vi "NXT_HINDBRAIN Move Motors.vi"(0 "NXT":T3, 1 "Motor Disable":bool, 2 "Tugboat Properties":T1={"_name"="Enterprise", "_pitch"=440, "_rudderCenter"=1450, "_propCenter"=1000, "_irServoCenter"=1000, "_rudderMin"=1450, "_rudderMax"=1450, "_propMin"=1000, "_propMax"=1000, "_irServoMin"=1000, "_irServoMax"=1000}, 3 "_motorData":T2) -> ()   [LabVIEW 2012, in "Tugboat.lvrbt"]
uses:
  Tugboat.lvrbt
  <vilib>/NXT/Subs/LVHSConnector.ctl
  motorData_t.ctl
  tugProperties_t.ctl
  <vilib>/NXT/Block Support/NXT_InputPort.ctl
  <vilib>/NXT/Dual Mode Library/prims/inRangeAndCoerce/inRangeAndCoerce_int.vi
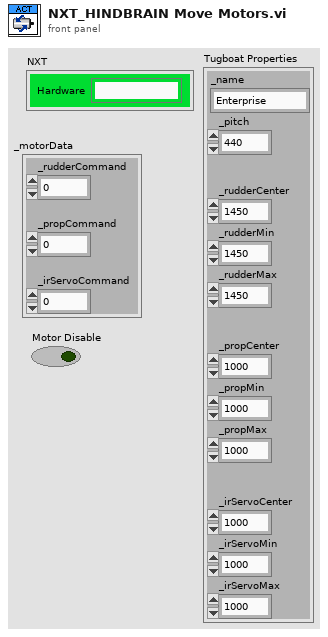
[diagram p1: front panel]
types:
  T1 = typedef "tugProperties_t.ctl" = cluster{"_name":string, "_pitch":i32, "_rudderCenter":u16, "_propCenter":u16, "_irServoCenter":u16, "_rudderMin":u16, "_rudderMax":u16, "_propMin":u16, "_propMax":u16, "_irServoMin":u16, "_irServoMax":u16}
  T2 = typedef "motorData_t.ctl" = cluster{"_rudderCommand":u16, "_propCommand":u16, "_irServoCommand":u16}
  T3 = typedef "LVHSConnector.ctl" = cluster{"Hardware":string, "Flattened String":string}
  T4 = cluster{"Servo Number":u8, "Position":u16, "Speed":u8}
  T5 = typedef "NXT_InputPort.ctl" = u8
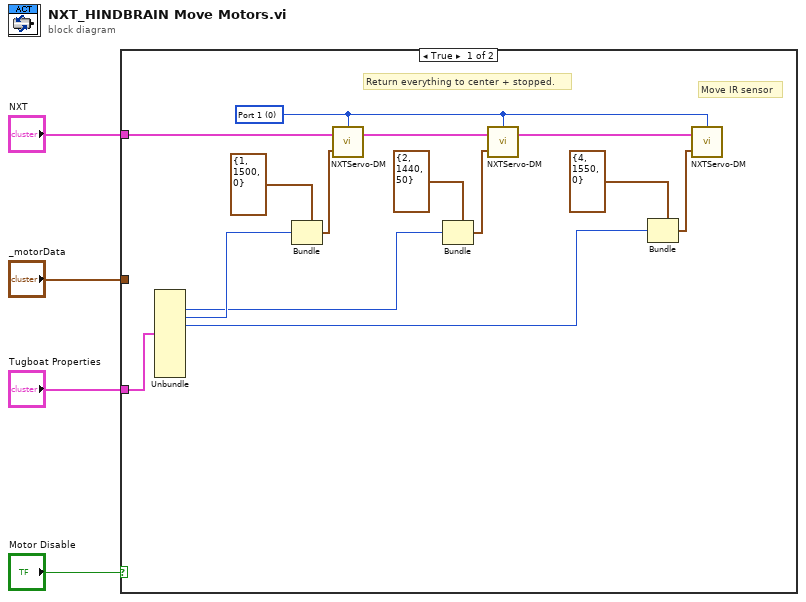
[diagram p0: block diagram]
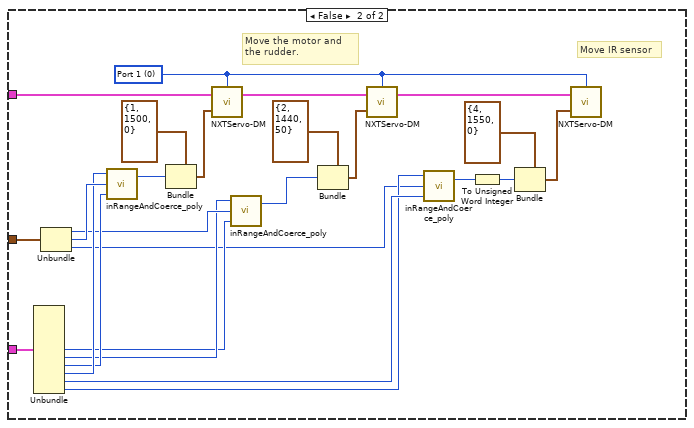
[diagram p2: hidden frame]
diagram:
  n1 = case shown="True" "Motor Disable" {
    tunnel: "NXT" -> [w15 w36]
    tunnel: "_motorData" -> [_ w35]
    tunnel: "Tugboat Properties" -> [w13 w31]
    frame True {
      w16 = T5 0 items=["Port 1", "Port 2", "Port 3", "Port 4"] ("Input Port")
      # "Move IR sensor"
      # "Return everything to center + stopped."
      n2 = Unbundle(w13) -> ("_rudderCenter"=w8:u16, "_propCenter"=w12:u16, "_irServoCenter"=w5:u16)  [unwired: 8 out]
      n3 = Bundle(cluster=T4 {"Servo Number"=1, "Position"=1500, "Speed"=0} ("Input of NXTServo"), "Position"=w12) -> (w11:T4)  [unwired: 2 in]
      n4 = call "NXTServo-DM.vi"("Input of NXTServo"=w11, "NXT"=w15, "Input Port"=w16) -> ("NXT dup"=w18:T3)  [unwired: 1 out]
      n5 = Bundle(cluster=T4 {"Servo Number"=2, "Position"=1440, "Speed"=50} ("Input of NXTServo"), "Position"=w8) -> (w9:T4)  [unwired: 2 in]
      n6 = call "NXTServo-DM.vi"("Input of NXTServo"=w9, "NXT"=w18, "Input Port"=w16) -> ("NXT dup"=w17:T3)  [unwired: 1 out]
      n7 = Bundle(cluster=T4 {"Servo Number"=4, "Position"=1550, "Speed"=0} ("Input of NXTServo"), "Position"=w5) -> (w7:T4)  [unwired: 2 in]
      n8 = call "NXTServo-DM.vi"("Input of NXTServo"=w7, "NXT"=w17, "Input Port"=w16) -> ()  [unwired: 2 out]
    }
    frame False {
      w33 = T5 0 items=["Port 1", "Port 2", "Port 3", "Port 4"] ("Input Port")
      # "Move IR sensor"
      # "Move the motor and \nthe rudder."
      n9 = Unbundle(w31) -> ("_rudderMin"=w23:u16, "_rudderMax"=w24:u16, "_propMin"=w27:u16, "_propMax"=w28:u16, "_irServoMin"=w21:u16, "_irServoMax"=w20:u16)  [unwired: 5 out]
      n10 = Unbundle(w35) -> ("_rudderCommand"=w26:u16, "_propCommand"=w30:u16, "_irServoCommand"=w19:u16)
      n11 = call-poly <vilib>:"inRangeAndCoerce_poly.vi"("lower limit"=w27, "x"=w30, "upper limit"=w28) -> ("coerced(x)"=w29:i32)  [unwired: 1 out]
      n12 = Bundle(cluster=T4 {"Servo Number"=1, "Position"=1500, "Speed"=0} ("Input of NXTServo"), "Position"=w29) -> (w40:T4)  [unwired: 2 in]
      n13 = call "NXTServo-DM.vi"("Input of NXTServo"=w40, "NXT"=w36, "Input Port"=w33) -> ("NXT dup"=w39:T3)  [unwired: 1 out]
      n14 = call-poly <vilib>:"inRangeAndCoerce_poly.vi"("lower limit"=w23, "x"=w26, "upper limit"=w24) -> ("coerced(x)"=w25:i32)  [unwired: 1 out]
      n15 = Bundle(cluster=T4 {"Servo Number"=2, "Position"=1440, "Speed"=50} ("Input of NXTServo"), "Position"=w25) -> (w43:T4)  [unwired: 2 in]
      n16 = call "NXTServo-DM.vi"("Input of NXTServo"=w43, "NXT"=w39, "Input Port"=w33) -> ("NXT dup"=w34:T3)  [unwired: 1 out]
      n17 = call-poly <vilib>:"inRangeAndCoerce_poly.vi"("lower limit"=w21, "x"=w19, "upper limit"=w20) -> ("coerced(x)"=w22:i32)  [unwired: 1 out]
      n18 = To Unsigned Word Integer(number=w22) -> (unsigned 16bit integer=w32:u16)
      n19 = Bundle(cluster=T4 {"Servo Number"=4, "Position"=1550, "Speed"=0} ("Input of NXTServo"), "Position"=w32) -> (w38:T4)  [unwired: 2 in]
      n20 = call "NXTServo-DM.vi"("Input of NXTServo"=w38, "NXT"=w34, "Input Port"=w33) -> ()  [unwired: 2 out]
    }
  }
